vi "Take_bck.vi"(7 "batch_bck location (should be on Desktop)":path, 9 "Number of Accumulations":i32, 10 "Exposure Time (s)":dbl format="%#_13g", 11 "Take_bck_scan.exe location":path) -> ()   [LabVIEW 2017]
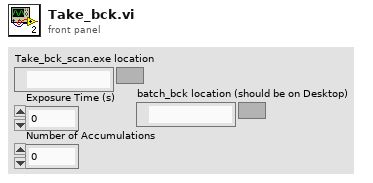
[diagram p1: front panel]
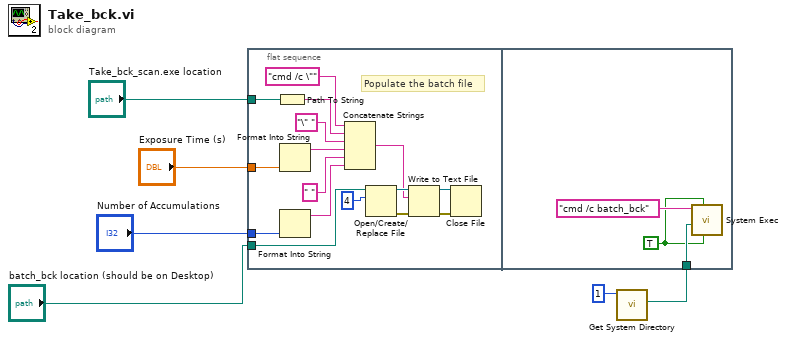
[diagram p0: block diagram]
diagram:
  n1 = flat-sequence {
    tunnel: "Exposure Time (s)" -> [w12]
    tunnel: "Number of Accumulations" -> [w13]
    tunnel: "batch_bck location (should be on Desktop)" -> [w22]
    tunnel: "Take_bck_scan.exe location" -> [w16]
    tunnel: w1 -> [w24]
    frame #0 {
      # "Populate the batch file"
      n2 = Path To String(path=w16) -> (string=w15:string)
      n3 = Format Into String(w12) -> (resulting string=w11:string)  [unwired: 3 in, 1 out]
      n4 = Format Into String(w13) -> (resulting string=w10:string)  [unwired: 3 in, 1 out]
      n5 = Concatenate Strings("cmd /c \"", w15, "\" ", w11, " ", w10) -> (w9:string)
      n6 = Open/Create/Replace File(file path (use dialog)=w22, operation (0:open)=4) -> (refnum out=w21:refnum<file>, error out=w20:errorcluster)  [unwired: 4 in, 1 out]
      n7 = Write to Text File(file (use dialog)=w21, text=w9, error in=w20) -> (refnum out=w18:refnum<file>, error out=w19:errorcluster)  [unwired: 1 in, 1 out]
      n8 = Close File(refnum=w18, error in=w19) -> ()  [unwired: 2 out]
    }
    frame #1 {
      w23 = TRUE
      n9 = call <vilib>:"System Exec.vi"("run minimized? (F)"=w23, "wait until completion? (T)"=w23, "working directory"=w24, "command line"="cmd /c batch_bck") -> ()  [unwired: 4 in, 4 out]
    }
  }
  n10 = call <vilib>:"Get System Directory.vi"("system directory type"=1) -> ("system directory"=w1:path)  [unwired: 10 in]
